vi "Draw Scan Frame Outline.vi"() -> ()   [LabVIEW 2021]
doc: "This example draws the outline of the current scan frame in the scan control module with a simple click. It gives also the option to add a mark at the current tip position.\n\nThe marks remain in the scan control module until programmatically erasing them with the corresponding functions.\n\n- Nanonis Programming Interface -"
uses:
  Nanonis Prog Interface.lvlib
panel:
  in  "Draw point":bool
  in  "Draw outline":bool
  in  "Clear last point":bool
  in  "Clear last outline":bool
  in  "Clear All":bool
  in  "Pen Color":u32(colorbox)=3381759
  in  "stop":bool
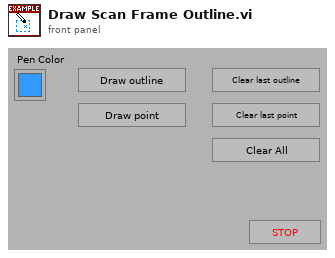
[diagram p1: front panel]
types:
  T1 = cluster{"Start":cluster{"X1 (m)":sgl, "Y1 (m)":sgl}, "End":cluster{"X2 (m)":sgl, "Y2 (m)":sgl}, "Line Color":u32, "Visible":bool}[]
  T2 = cluster{"X (m)":sgl, "Y (m)":sgl, "Text":string, "Color":u32, "Visible":bool}[]
  T3 = cluster{"Xc":sgl, "Yc":sgl, "Width":sgl, "Height":sgl, "Angle (deg)":sgl}
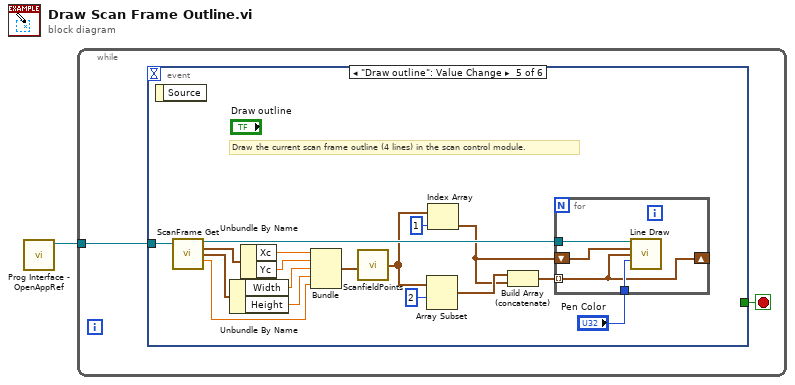
[diagram p0: block diagram]
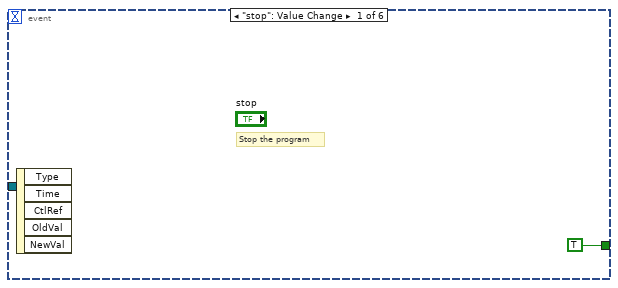
[diagram p2: hidden frame]
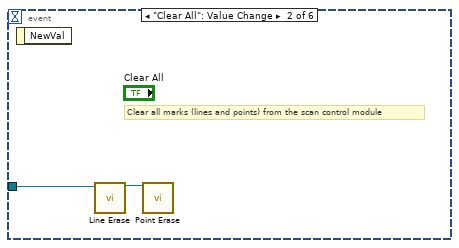
[diagram p3: hidden frame]
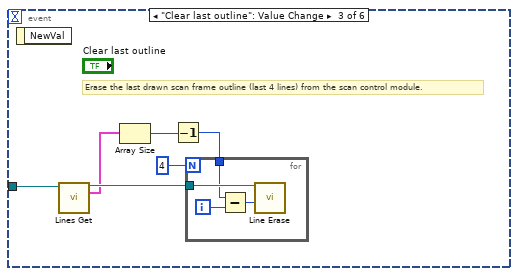
[diagram p4: hidden frame]
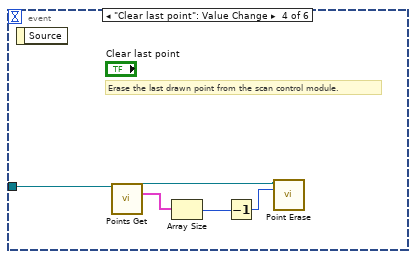
[diagram p5: hidden frame]
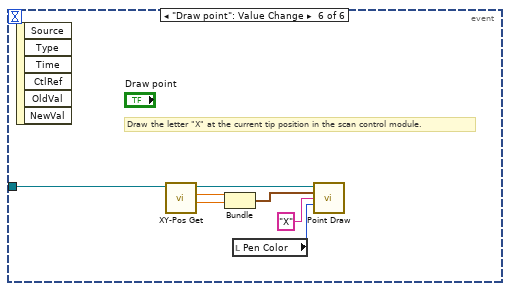
[diagram p6: hidden frame]
diagram:
  n1 = call <userlib>:"Prog Interface - OpenAppRef.vi"() -> ("Application reference"=w1:refnum<vi>)  [unwired: 6 in, 1 out]
  n2 = while {
    tunnel: w1 -> [w2]
    stop <- w3 stop-if-true
    n3 = event shown="[4] \"Draw outline\": Value Change" {
      selector: _ -> [_ _ _ _ _ _]
      dyn-events: _ -> [_ _ _ _ _ _]
      timeout: _ -> [_ _ _ _ _ _]
      tunnel: [TRUE ("stop") _ _ _ _ _] -> w3
      tunnel: w2 -> [_ w6 w12 w21 w38 w49]
      event "stop": Value Change {
        # "Stop the program"
        n4 = event-data() -> ()  [unwired: 1 in, 5 out]
      }
      event "Clear All": Value Change {
        # "Clear all marks (lines and points) from the scan control module"
        n5 = event-data() -> ()  [unwired: 1 in, 1 out]
        n6 = call <userlib>:"Line Erase.vi"("Application ref in"=w6) -> ("Application ref out"=w5:refnum<vi>)  [unwired: 13 in, 1 out]
        n7 = call <userlib>:"Point Erase.vi"("Application ref in"=w5) -> ()  [unwired: 13 in, 2 out]
      }
      event "Clear last outline": Value Change {
        # "Erase the last drawn scan frame outline (last 4 lines) from the scan control module."
        n8 = event-data() -> ()  [unwired: 1 in, 1 out]
        n9 = call <userlib>:"Lines Get.vi"("Application ref in"=w12) -> ("Application ref out"=w11:refnum<vi>, "Lines"=w10:T1)  [unwired: 12 in, 1 out]
        n10 = Array Size(array=w10) -> (size(s)=w8:i32)
        n11 = Decrement(x=w8) -> (x-1=w7:i32)
        n12 = for {
          N: 4 -> [_]
          tunnel: w11 -> [w16]
          tunnel: w7 -> [w15]
          i -> [w14]
          n13 = Subtract(x=w15, y=w14) -> (x-y=w13:i32)
          n14 = call <userlib>:"Line Erase.vi"("Application ref in"=w16, "Line index (-1=All lines)"=w13) -> ()  [unwired: 12 in, 2 out]
        }
      }
      event "Clear last point": Value Change {
        # "Erase the last drawn point from the scan control module."
        n15 = event-data() -> ()  [unwired: 1 in, 1 out]
        n16 = call <userlib>:"Points Get.vi"("Application ref in"=w21) -> ("Application ref out"=w19:refnum<vi>, "Points"=w20:T2)  [unwired: 12 in, 1 out]
        n17 = Array Size(array=w20) -> (size(s)=w17:i32)
        n18 = Decrement(x=w17) -> (x-1=w18:i32)
        n19 = call <userlib>:"Point Erase.vi"("Application ref in"=w19, "Point index (-1=All points)"=w18) -> ()  [unwired: 12 in, 2 out]
      }
      event "Draw outline": Value Change {
        # "Draw the current scan frame outline (4 lines) in the scan control module."
        n20 = event-data() -> ()  [unwired: 1 in, 1 out]
        n21 = call <userlib>:"ScanFrame Get.vi"("Application ref in"=w38) -> ("Application ref out"=w37:refnum<vi>, "Center coordinates (m)"=w35:cluster{"Xc":sgl, "Yc":sgl}, "Size (m)"=w34:cluster{"Width":sgl, "Height":sgl}, "Angle (deg)"=w29:sgl)  [unwired: 10 in, 1 out]
        n22 = Unbundle By Name(w34) -> ("Width"=w31:sgl, "Height"=w30:sgl)
        n23 = Unbundle By Name(w35) -> ("Xc"=w33:sgl, "Yc"=w32:sgl)
        n24 = Bundle("Xc"=w33, "Yc"=w32, "Width"=w31, "Height"=w30, "Angle (deg)"=w29) -> (w28:T3)  [unwired: 1 in]
        n25 = call <userlib>:"ScanfieldPoints.vi"("Scanfield"=w28) -> ("points"=w26:cluster{"X (m)":sgl, "Y (m)":sgl}[])  [unwired: 4 in]
        n26 = Array Subset(array=w26, index=2) -> (w24:cluster{"X (m)":sgl, "Y (m)":sgl}[])  [unwired: 1 in]
        n27 = Index Array(array=w26, index=1) -> (element=w23:cluster{"X (m)":sgl, "Y (m)":sgl})
        n28 = Build Array (concatenate)(w24, w23) -> (w22:cluster{"X (m)":sgl, "Y (m)":sgl}[])
        n29 = for {
          tunnel: w37 -> [w42]
          shift-right: [w39] -> _
          shift-left: w23 -> [w41]
          tunnel: w22 -> [w39] mode=indexing
          tunnel: "Pen Color" -> [w40]
          n30 = call <userlib>:"Line Draw.vi"("Application ref in"=w42, "Start Point Coordinates"=w41, "End Point Coordinates"=w39, "Color"=w40) -> ()  [unwired: 10 in, 2 out]
        }
      }
      event "Draw point": Value Change {
        # "Draw the letter \"X\" at the current tip position in the scan control module."
        n31 = event-data() -> ()  [unwired: 1 in, 6 out]
        n32 = call <userlib>:"XY-Pos Get.vi"("Application ref in"=w49) -> ("Y (m)"=w44:sgl, "X (m)"=w45:sgl, "Application ref out"=w48:refnum<vi>)  [unwired: 6 in, 1 out]
        n33 = Bundle("X (m)"=w45, "Y (m)"=w44) -> (w43:cluster{"X (m)":sgl, "Y (m)":sgl})  [unwired: 1 in]
        n34 = local read "Pen Color"() -> (w47:u32)
        n35 = call <userlib>:"Point Draw.vi"("Application ref in"=w48, "Point Coordinates"=w43, "Text"="X", "Color"=w47) -> ()  [unwired: 10 in, 2 out]
      }
    }
  }
